vi "Sub_interpolate.vi"   [LabVIEW 2021]
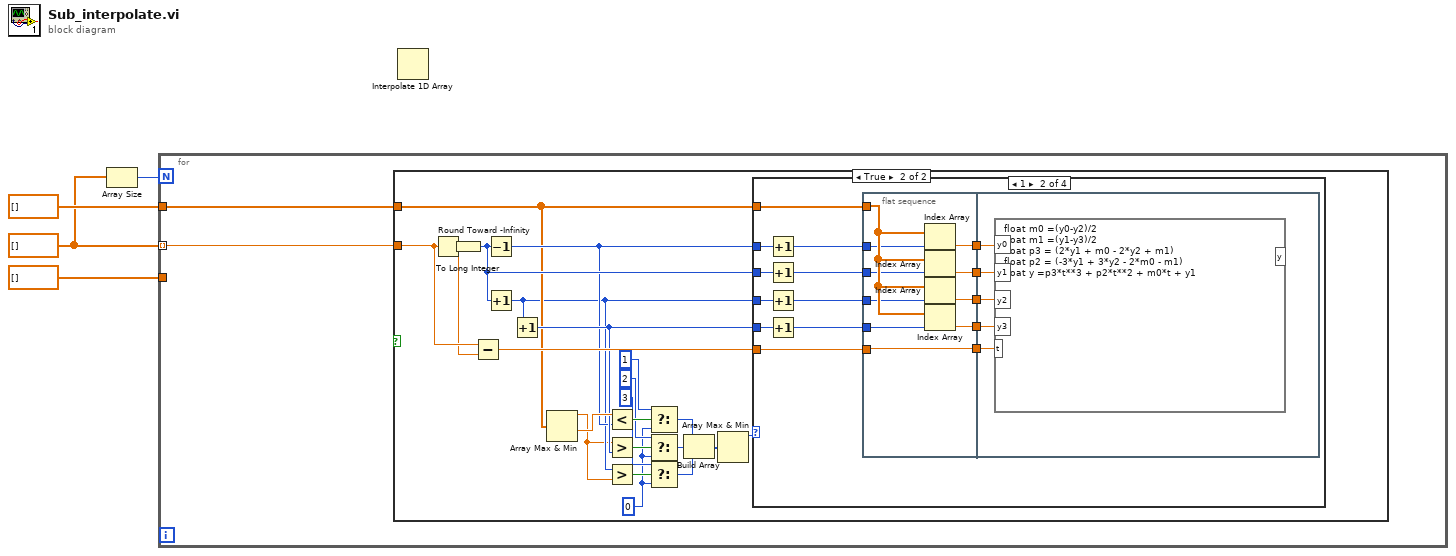
[diagram p0: block diagram]
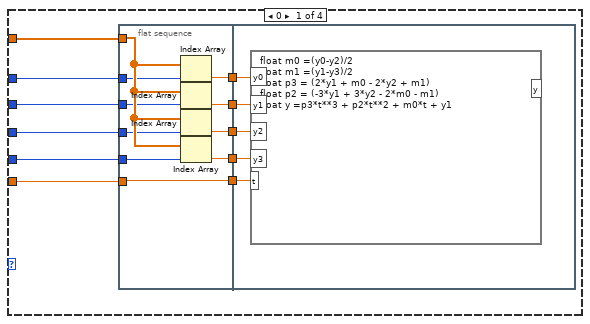
[diagram p3: hidden frame]
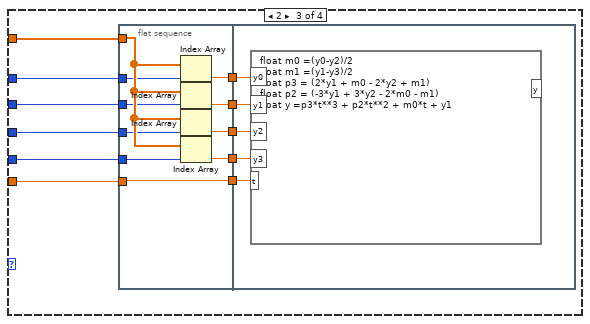
[diagram p4: hidden frame]
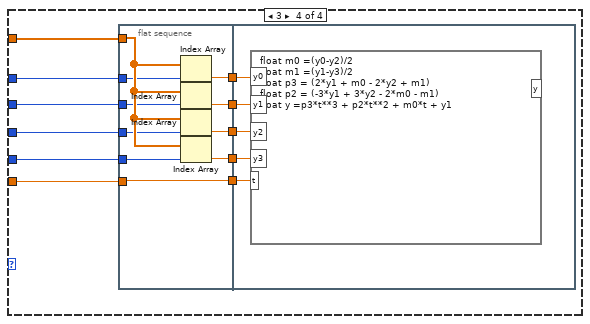
[diagram p5: hidden frame]
diagram:
  w2 = dbl[] []
  n1 = Array Size(array=w2) -> (size(s)=w3:i32)
  n2 = for {
    N: w3 -> [_]
    tunnel: dbl[] [] -> [w5]
    tunnel: w2 -> [w6] mode=indexing
    tunnel: dbl[] [] -> [_]
    n3 = case shown="True" {
      selector: _ -> [_ _]
      tunnel: w6 -> [_ w27]
      tunnel: w5 -> [_ w19]
      frame False {
      }
      frame True {
        w7 = 0 ("f")
        n4 = Round Toward -Infinity(1:w27) -> (0:w26:dbl)
        n5 = To Long Integer(number=w26) -> (32bit integer=w25:i32)
        n6 = Subtract(x=w27, y=w26) -> (x-y=w28:dbl)
        n7 = Decrement(x=w25) -> (x-1=w22:i32)
        n8 = Increment(x=w25) -> (x+1=w11:i32)
        n9 = Increment(x=w11) -> (x+1=w23:i32)
        n10 = Array Max & Min(array=w19) -> (max value=w10:dbl, min value=w24:dbl)  [unwired: 2 out]
        n11 = Less?(x=w24, y=w22) -> (x < y?=w21:bool)
        n12 = Greater?(x=w10, y=w23) -> (0:w20:bool)
        n13 = Greater?(x=w11, y=w10) -> (0:w12:bool)
        n14 = Select(t=1, s=w21, f=w7) -> (s? t:f=w16:i32)
        n15 = Select(t=2, s=w20, f=w7) -> (s? t:f=w15:i32)
        n16 = Select(t=3, s=w12, f=w7) -> (s? t:f=w8:i32)
        n17 = Build Array(w16, w15, w8) -> (w14:i32[])
        n18 = Array Max & Min(array=w14) -> (max value=w13:i32)  [unwired: 3 out]
        n19 = case shown="1" w13 {
          tunnel: w19 -> [w34 w64 w90 w116]
          tunnel: w28 -> [w33 w63 w89 w115]
          tunnel: w23 -> [w32 w62 w88 w114]
          tunnel: w11 -> [w31 w61 w87 w113]
          tunnel: w22 -> [w30 w60 w86 w112]
          tunnel: w25 -> [w29 w59 w85 w111]
          frame 0 {
            n20 = flat-sequence {
              tunnel: [w48] -> w39
              tunnel: [w47] -> w38
              tunnel: [w46] -> w37
              tunnel: [w45] -> w36
              tunnel: [w44] -> w35
              tunnel: w34 -> [w49]
              tunnel: w33 -> [w48]
              tunnel: w32 -> [w43]
              tunnel: w31 -> [w42]
              tunnel: w30 -> [w41]
              tunnel: w29 -> [w40]
              tunnel: w39 -> [w54]
              tunnel: w38 -> [w53]
              tunnel: w37 -> [w52]
              tunnel: w36 -> [w51]
              tunnel: w35 -> [w50]
              frame #0 {
                n21 = Index Array(array=w49, index=w41) -> (element=w47:dbl)
                n22 = Index Array(array=w49, index=w40) -> (element=w46:dbl)
                n23 = Index Array(array=w49, index=w42) -> (element=w45:dbl)
                n24 = Index Array(array=w49, index=w43) -> (element=w44:dbl)
              }
              frame #1 {
                n25 = formula code="float m0 =(y0-y2)/2\nfloat m1 =(y1-y3)/2\nfloat p3 = (2*y1 + m0 - 2*y2 + m1)\nfloat p2 = (-3*y1 + 3*y2 - 2*m0 - m1)\nfloat y =p3*t**3 + p2*t**2 + m0*t + y1"("y0"=w53, "y1"=w52, "y2"=w51, "y3"=w50, "t"=w54) -> ()  [unwired: 1 out]
              }
            }
          }
          frame 1 {
            n26 = Increment(x=w60) -> (x+1=w58:i32)
            n27 = Increment(x=w59) -> (x+1=w57:i32)
            n28 = Increment(x=w61) -> (x+1=w56:i32)
            n29 = Increment(x=w62) -> (x+1=w55:i32)
            n30 = flat-sequence {
              tunnel: [w78] -> w69
              tunnel: [w77] -> w68
              tunnel: [w76] -> w67
              tunnel: [w75] -> w66
              tunnel: [w74] -> w65
              tunnel: w64 -> [w79]
              tunnel: w63 -> [w78]
              tunnel: w55 -> [w73]
              tunnel: w56 -> [w72]
              tunnel: w58 -> [w71]
              tunnel: w57 -> [w70]
              tunnel: w69 -> [w84]
              tunnel: w68 -> [w83]
              tunnel: w67 -> [w82]
              tunnel: w66 -> [w81]
              tunnel: w65 -> [w80]
              frame #0 {
                n31 = Index Array(array=w79, index=w71) -> (element=w77:dbl)
                n32 = Index Array(array=w79, index=w70) -> (element=w76:dbl)
                n33 = Index Array(array=w79, index=w72) -> (element=w75:dbl)
                n34 = Index Array(array=w79, index=w73) -> (element=w74:dbl)
              }
              frame #1 {
                n35 = formula code="float m0 =(y0-y2)/2\nfloat m1 =(y1-y3)/2\nfloat p3 = (2*y1 + m0 - 2*y2 + m1)\nfloat p2 = (-3*y1 + 3*y2 - 2*m0 - m1)\nfloat y =p3*t**3 + p2*t**2 + m0*t + y1"("y0"=w83, "y1"=w82, "y2"=w81, "y3"=w80, "t"=w84) -> ()  [unwired: 1 out]
              }
            }
          }
          frame 2 {
            n36 = flat-sequence {
              tunnel: [w104] -> w95
              tunnel: [w103] -> w94
              tunnel: [w102] -> w93
              tunnel: [w101] -> w92
              tunnel: [w100] -> w91
              tunnel: w90 -> [w105]
              tunnel: w89 -> [w104]
              tunnel: w88 -> [w99]
              tunnel: w87 -> [w98]
              tunnel: w86 -> [w97]
              tunnel: w85 -> [w96]
              tunnel: w95 -> [w110]
              tunnel: w94 -> [w109]
              tunnel: w93 -> [w108]
              tunnel: w92 -> [w107]
              tunnel: w91 -> [w106]
              frame #0 {
                n37 = Index Array(array=w105, index=w97) -> (element=w103:dbl)
                n38 = Index Array(array=w105, index=w96) -> (element=w102:dbl)
                n39 = Index Array(array=w105, index=w98) -> (element=w101:dbl)
                n40 = Index Array(array=w105, index=w99) -> (element=w100:dbl)
              }
              frame #1 {
                n41 = formula code="float m0 =(y0-y2)/2\nfloat m1 =(y1-y3)/2\nfloat p3 = (2*y1 + m0 - 2*y2 + m1)\nfloat p2 = (-3*y1 + 3*y2 - 2*m0 - m1)\nfloat y =p3*t**3 + p2*t**2 + m0*t + y1"("y0"=w109, "y1"=w108, "y2"=w107, "y3"=w106, "t"=w110) -> ()  [unwired: 1 out]
              }
            }
          }
          frame 3 {
            n42 = flat-sequence {
              tunnel: [w130] -> w121
              tunnel: [w129] -> w120
              tunnel: [w128] -> w119
              tunnel: [w127] -> w118
              tunnel: [w126] -> w117
              tunnel: w116 -> [w131]
              tunnel: w115 -> [w130]
              tunnel: w114 -> [w125]
              tunnel: w113 -> [w124]
              tunnel: w112 -> [w123]
              tunnel: w111 -> [w122]
              tunnel: w121 -> [w136]
              tunnel: w120 -> [w135]
              tunnel: w119 -> [w134]
              tunnel: w118 -> [w133]
              tunnel: w117 -> [w132]
              frame #0 {
                n43 = Index Array(array=w131, index=w123) -> (element=w129:dbl)
                n44 = Index Array(array=w131, index=w122) -> (element=w128:dbl)
                n45 = Index Array(array=w131, index=w124) -> (element=w127:dbl)
                n46 = Index Array(array=w131, index=w125) -> (element=w126:dbl)
              }
              frame #1 {
                n47 = formula code="float m0 =(y0-y2)/2\nfloat m1 =(y1-y3)/2\nfloat p3 = (2*y1 + m0 - 2*y2 + m1)\nfloat p2 = (-3*y1 + 3*y2 - 2*m0 - m1)\nfloat y =p3*t**3 + p2*t**2 + m0*t + y1"("y0"=w135, "y1"=w134, "y2"=w133, "y3"=w132, "t"=w136) -> ()  [unwired: 1 out]
              }
            }
          }
        }
      }
    }
  }
  n48 = Interpolate 1D Array() -> ()  [unwired: 2 in, 1 out]
